vi "DTACQ - Write List of Commands to Text File.vi"(8 "error in":errorcluster, 9 "File Path":path, 10 "Port":u16, 11 "Address":string) -> (0 "error out":errorcluster)   [LabVIEW 2017, in "Communications Library.lvlib"]
doc: "Saves a list of avilable commands to a tab seperated values file.\n\nThe \"help\" command is used to retrieve the list of commands."
uses:
  Communications Library.lvlib
  <vilib>/Utility/file.llb/Write Delimited Spreadsheet (string).vi
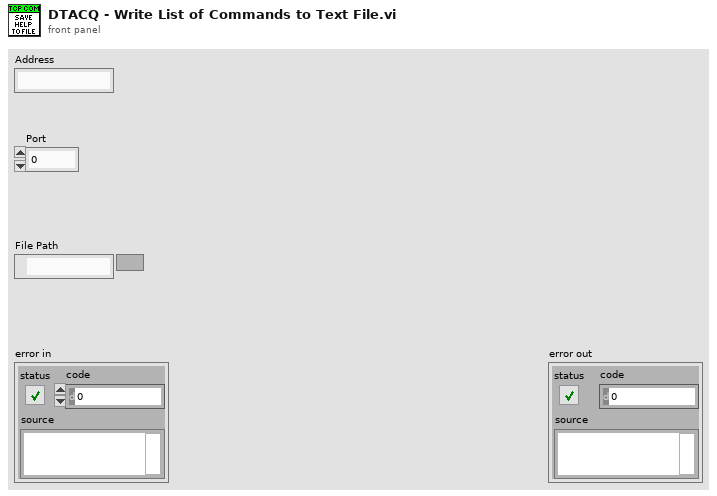
[diagram p1: front panel]
types:
  T1 = typedef "Communications Library.lvlib/DTACQ Connection Data--Cluster.ctl" = cluster{"Description":string, "Address":string, "Port":u16, "timeout (ms)":i32, "Termination Character":string, "TCP Connection Reference":refnum<k5>, "Open Connection":bool}
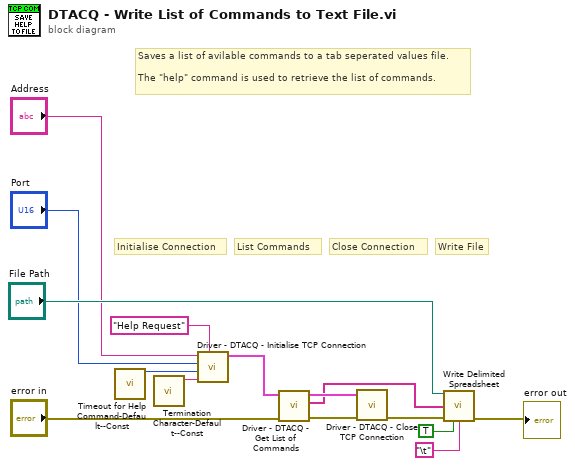
[diagram p0: block diagram]
diagram:
  # "Write File"
  # "Close Connection"
  # "List Commands"
  # "Initialise Connection"
  # "Saves a list of avilable commands to a tab seperated values file.\n\nThe \"help\" command is used to retrieve the list of commands."
  n1 = call "Timeout for Help Command-Default--Const.vi"() -> ("timeout (ms)"=w2:i32)  [unwired: 11 in]
  n2 = call "Termination Character-Default--Const.vi"() -> ("Termination Character"=w1:string)  [unwired: 11 in]
  n3 = call "Driver - DTACQ - Initialise TCP Connection.vi"("Description"="Help Request", "Termination Character"=w1, "timeout (ms)"=w2, "Port"="Port", "Address"="Address") -> ("DTACQ Connection Data Out"=w7:T1)  [unwired: 6 in]
  n4 = call "Driver - DTACQ - Get List of Commands.vi"("error in"="error in", "DTACQ Connection Data In"=w7) -> ("error out"=w10:errorcluster, "Commands"=w9:string[], "DTACQ Connection Data Out"=w11:T1)  [unwired: 7 in]
  n5 = call "Driver - DTACQ - Close TCP Connection.vi"("error in"=w10, "DTACQ Connection Data In"=w11) -> ("error out"=w8:errorcluster)  [unwired: 8 in, 1 out]
  n6 = call-poly <vilib>:"Write Delimited Spreadsheet.vi"("file path (dialog if empty)"="File Path", "1D data"=w9, "error in (no error)"=w8, "transpose? (no:F)"=TRUE, "delimiter (\\t)"="\t") -> ("error out"=→"error out":errorcluster)  [unwired: 9 in, 1 out]
